vi "getRange.vi"(8 "error in (no error)":errorcluster, 11 "Electrometer in":refnum<class "Electrometer.lvclass">) -> (0 "error out":errorcluster, 2 "Range":string, 3 "Electrometer out":refnum<class "Electrometer.lvclass">)   [LabVIEW 2016, in "Electrometer.lvclass"]
uses:
  Electrometer.lvclass
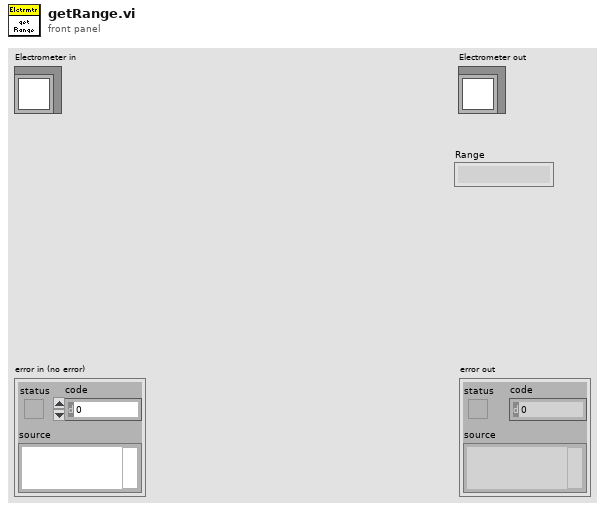
[diagram p1: front panel]
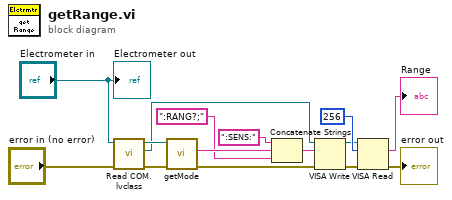
[diagram p0: block diagram]
diagram:
  n1 = call "Read COM.lvclass.vi"("error in (no error)"="error in (no error)", "Electrometer in"="Electrometer in") -> ("error out"=w14:errorcluster, "VISA"=w8:refnum<visa-resource-name>, "Electrometer out"=w15:refnum<class "Electrometer.lvclass">)  [unwired: 7 in]
  n2 = call "getMode.vi"("error in (no error)"=w14, "Electrometer in"=w15) -> ("error out"=w7:errorcluster, "Mode"=w12:string)  [unwired: 7 in, 1 out]
  n3 = Concatenate Strings(":SENS:", w12, ":RANG?;" ("string")) -> (w6:string)
  n4 = VISA Write(VISA resource name=w8, write buffer=w6, error in (no error)=w7) -> (VISA resource name out=w3:refnum<visa-resource-name>, error out=w4:errorcluster)  [unwired: 1 out]
  n5 = VISA Read(VISA resource name=w3, byte count=u32 256, error in (no error)=w4) -> (read buffer=→"Range":string, error out=→"error out":errorcluster)  [unwired: 2 out]
  "Electrometer out" <- "Electrometer in"
